vi "Array booleano para Float (IEEE 754).vi"(1 "Array [32]":bool[](array[boolean])) -> (0 "Float [SGL]":sgl)   [LabVIEW 2019]
doc: "Recebe um array booleano com o seguinte formatato: [SINAL EXPOENTE MANTISSA]. O sinal tem apenas um bit (0 = positivo, 1 = negativo), o expoente tem oito bits (posição 1 a 8 no array) e a mantissa tem os outros 23 bits (posição 9 a 31 no array). A saída é um float (single) convertido segundo a convenção IEEE 754."
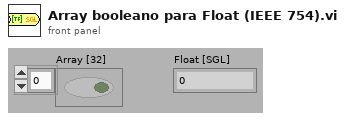
[diagram p1: front panel]
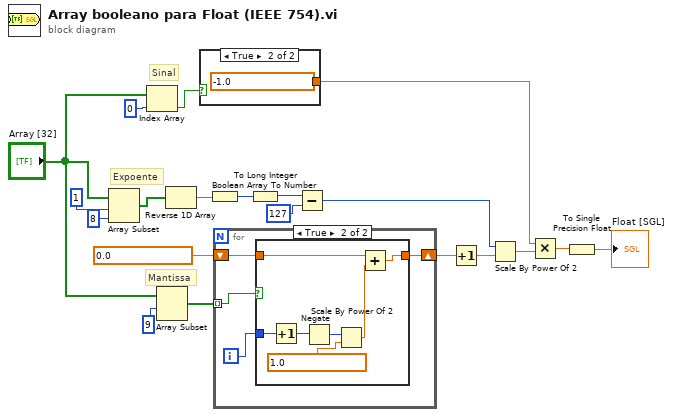
[diagram p0: block diagram]
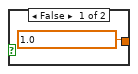
[diagram p2: hidden frame]
diagram:
  # "Mantissa"
  # "Expoente"
  # "Sinal"
  n1 = Array Subset(array="Array [32]", index=1, length=8) -> (w10:bool[])
  n2 = Index Array(array="Array [32]", index=0) -> (element=w9:bool)
  n3 = Array Subset(array="Array [32]", index=9) -> (w6:bool[])  [unwired: 1 in]
  n4 = Reverse 1D Array(array=w10) -> (reversed array=w11:bool[])
  n5 = case shown="True" w9 {
    tunnel: [1.0 -1.0] -> w17
    frame False {
    }
    frame True {
    }
  }
  n6 = Boolean Array To Number(Boolean array=w11) -> (number=w12:u32)
  n7 = for {
    shift-right: [w24] -> w7
    shift-left: 0.0 -> [w25]
    tunnel: w6 -> [w26] mode=indexing
    i -> [w23]
    n8 = case shown="True" w26 {
      tunnel: w25 -> [w27 w34]
      tunnel: [w27 w33] -> w24
      tunnel: w23 -> [_ w32]
      frame False {
      }
      frame True {
        n9 = Increment(x=w32) -> (x+1=w31:i32)
        n10 = Negate(x=w31) -> (-x=w30:i32)
        n11 = Scale By Power Of 2(n=w30, x=1.0) -> (x*2^n=w29:dbl)
        n12 = Add(x=w34, y=w29) -> (x+y=w33:dbl)
      }
    }
  }
  n13 = To Long Integer(number=w12) -> (32bit integer=w13:i32)
  n14 = Subtract(x=w13, y=127) -> (x-y=w15:i32)
  n15 = Increment(x=w7) -> (x+1=w8:dbl)
  n16 = Scale By Power Of 2(n=w15, x=w8) -> (x*2^n=w16:dbl)
  n17 = Multiply(x=w17, y=w16) -> (x*y=w18:dbl)
  n18 = To Single Precision Float(number=w18) -> (single precision float=→"Float [SGL]":sgl)
